vi "BRig_RT__Case_Exp__State_WrongOrTimeout_Pre__v11.vi"(0 "input_dataCurrent":u16[](array[numeric]), 5 "input_WorTO":bool, 6 "input_dataLC":u16[](array[numeric]), 7 "input_dataBlock":u16[][](array[numeric]), 9 "input_dataTrial":u16[][](array[numeric]), 11 "input_dataExp":u16[](array[numeric])) -> (1 "output_BTPR":bool, 2 "output_T2R":bool, 3 "output_T2R_or_BTPR":u16, 4 "output_dataCurrent":u16[](array[numeric]), 8 "output_dataBlock":u16[][](array[numeric]), 10 "output_dataTrial":u16[][](array[numeric]), 12 "output_BTPRavg":dbl, 13 "output_T2Ravg":dbl, 14 "output_R(F)_or_L(T)":bool, 15 "output_haveNewAvg":bool)   [LabVIEW 2014]
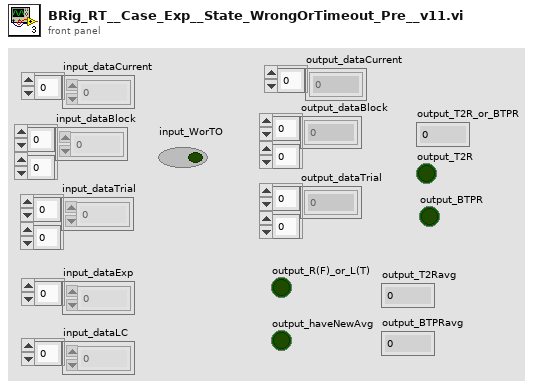
[diagram p1: front panel]
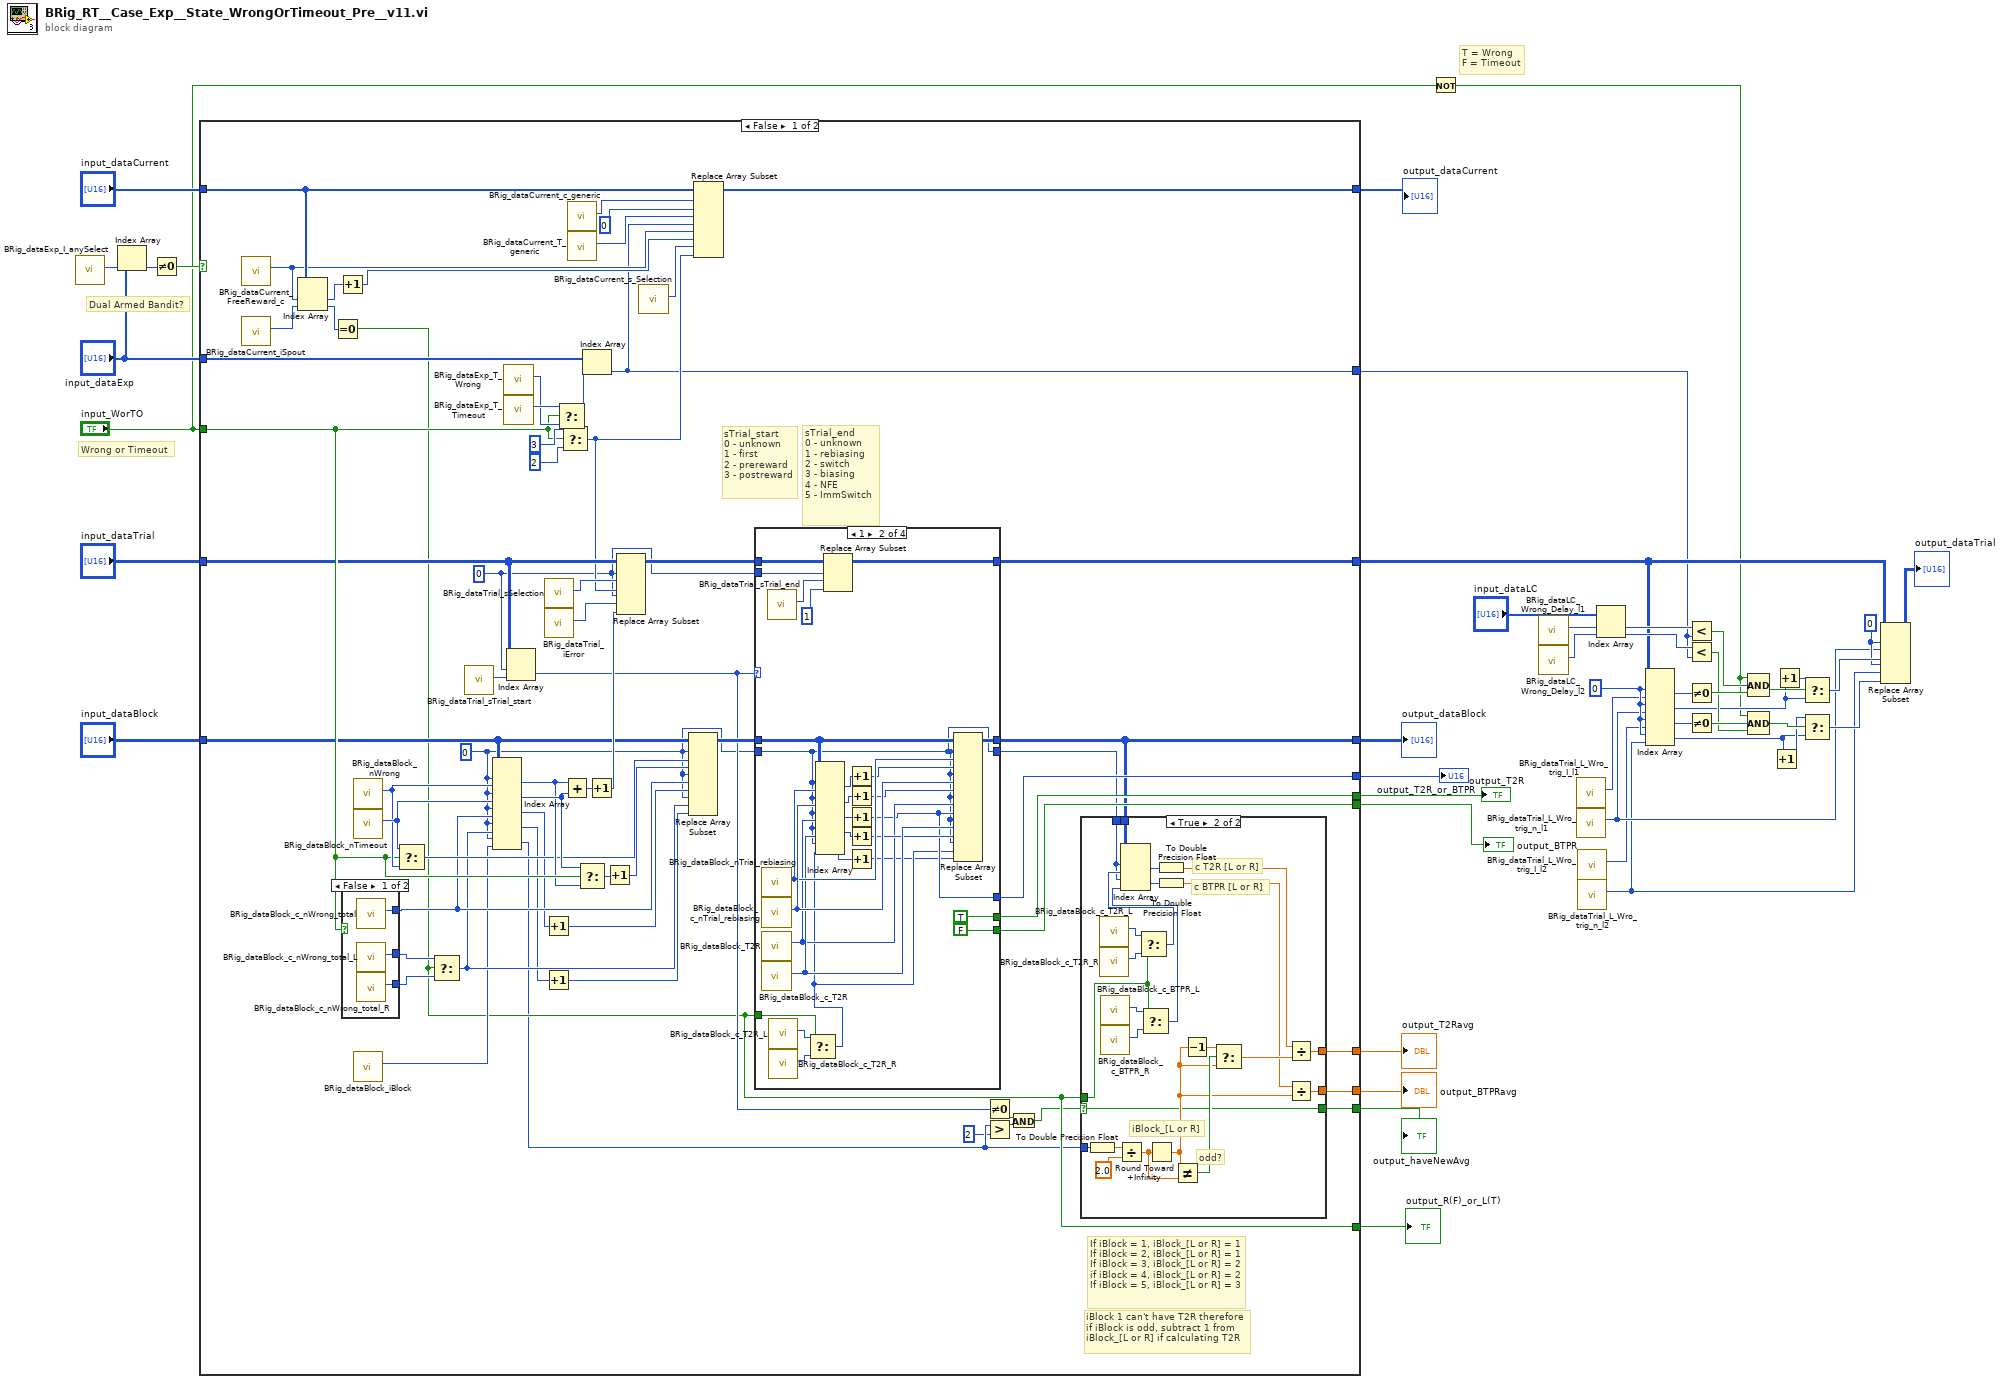
[diagram p0: block diagram]
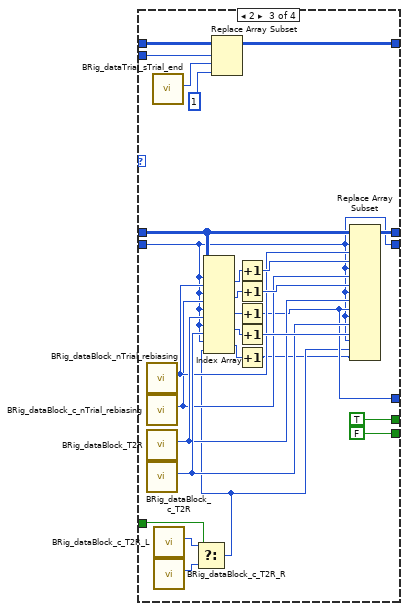
[diagram p4: hidden frame]
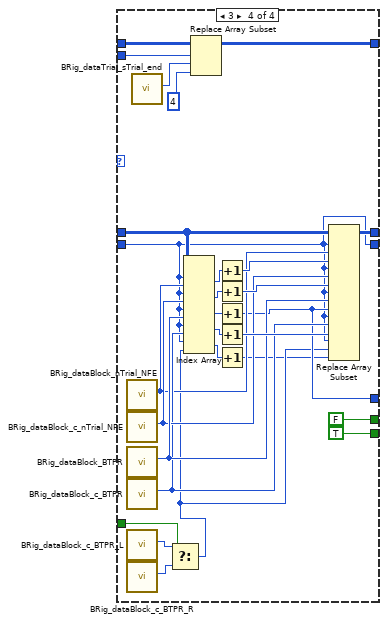
[diagram p5: hidden frame]
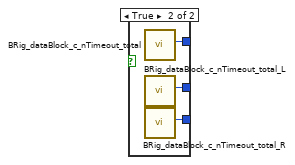
[diagram p6: hidden frame]
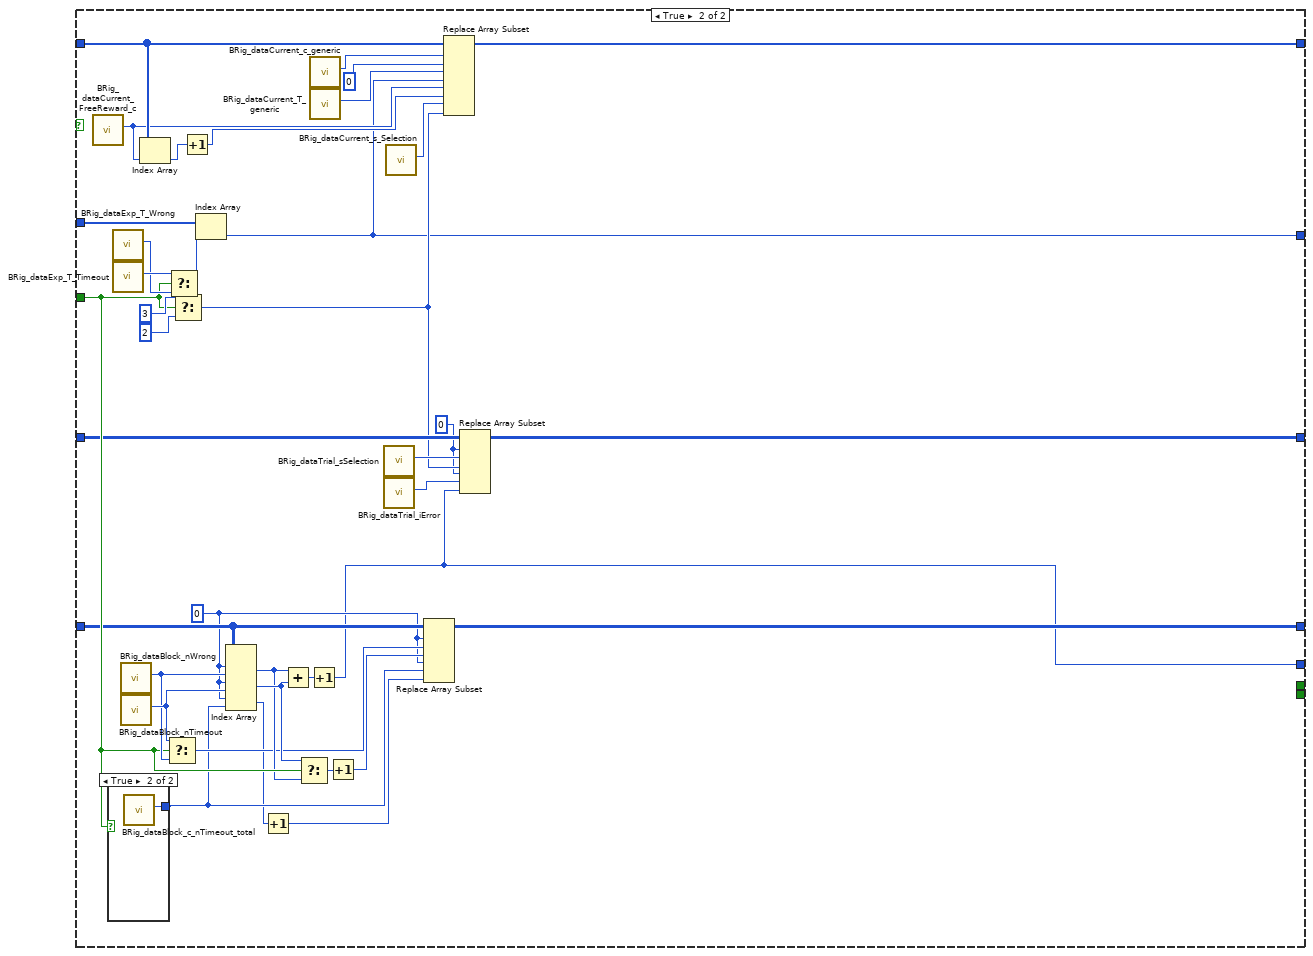
[diagram p7: hidden frame]
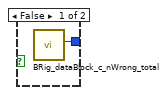
[diagram p8: hidden frame]
diagram:
  w17 = 0 ("index (row)")
  w27 = 0 ("disabled index (row)")
  # "T = Wrong\nF = Timeout"
  # "Wrong or Timeout"
  # "Dual Armed Bandit?"
  n1 = call "BRig_dataExp_I_anySelect.vi"() -> ("output_I_anySelect"=w34:i32)  [unwired: 11 in]
  n2 = Index Array(array="input_dataExp", index=w34) -> (element=w33:u16)
  n3 = Not Equal To 0?(x=w33) -> (x != 0?=w31:bool)
  n4 = case shown="False" w31 {
    tunnel: [w109 w264] -> w46
    tunnel: "input_dataCurrent" -> [w105 w260]
    tunnel: "input_dataExp" -> [w104 w259]
    tunnel: "input_WorTO" -> [w90 w248]
    tunnel: "input_dataBlock" -> [w86 w244]
    tunnel: "input_dataTrial" -> [w76 w238]
    tunnel: [w73 w231] -> w11
    tunnel: [w67 w228] -> w42
    tunnel: [w66 _] -> w41
    tunnel: [w65 _] -> w40
    tunnel: [w58 _] -> w39
    tunnel: [w57 w230] -> w38
    tunnel: [w55 _] -> w37
    tunnel: [w54 _] -> w36
    tunnel: [w53 _] -> w35
    tunnel: [w47 w227] -> w9
    frame False {
      w61 = 0
      w62 = 0
      # "iBlock 1 can't have T2R therefore\nif iBlock is odd, subtract 1 from\niBlock_[L or R] if calculating T2R"
      # "If iBlock = 1, iBlock_[L or R] = 1\nIf iBlock = 2, iBlock_[L or R] = 1\nIf iBlock = 3, iBlock_[L or R] = 2\nif iBlock = 4, iBlock_[L or R] = 2\nIf iBlock = 5, iBlock_[L or R] = 3"
      # "sTrial_end\n0 - unknown\n1 - rebiasing\n2 - switch\n3 - biasing\n4 - NFE\n5 - ImmSwitch"
      # "sTrial_start\n0 - unknown\n1 - first\n2 - prereward\n3 - postreward"
      n5 = call "BRig_dataCurrent_FreeReward_c.vi"() -> ("output_FreeReward_c"=w71:i32)  [unwired: 11 in]
      n6 = call "BRig_dataCurrent_iSpout.vi"() -> ("output_iSpout"=w60:i32)  [unwired: 11 in]
      n7 = Index Array(array=w105, index #1=w71, index #2=w60) -> (element #1=w72:u16, element #2=w59:u16)
      n8 = Equal To 0?(x=w59) -> (x = 0?=w58:bool)
      n9 = Increment(x=w72) -> (x+1=w70:u16)
      n10 = case shown="False" w90 {
        tunnel: [w223 w226] -> w83
        tunnel: [w222 w225] -> w96
        tunnel: [w221 w224] -> w95
        frame False {
          n11 = call "BRig_dataBlock_c_nWrong_total.vi"() -> ("output_c_nWrong_total"=w223:i32)  [unwired: 11 in]
          n12 = call "BRig_dataBlock_c_nWrong_total_L.vi"() -> ("output_c_nWrong_total_L"=w222:i32)  [unwired: 11 in]
          n13 = call "BRig_dataBlock_c_nWrong_total_R.vi"() -> ("output_c_nWrong_total_R"=w221:i32)  [unwired: 11 in]
        }
        frame True {
          n14 = call "BRig_dataBlock_c_nTimeout_total.vi"() -> ("output_c_nTimeout_total"=w226:i32)  [unwired: 11 in]
          n15 = call "BRig_dataBlock_c_nTimeout_total_L.vi"() -> ("output_c_nTimeout_total_L"=w225:i32)  [unwired: 11 in]
          n16 = call "BRig_dataBlock_c_nTimeout_total_R.vi"() -> ("output_c_nTimeout_total_R"=w224:i32)  [unwired: 11 in]
        }
      }
      n17 = call "BRig_dataBlock_nWrong.vi"() -> ("output_nWrong"=w91:i32)  [unwired: 11 in]
      n18 = call "BRig_dataBlock_nTimeout.vi"() -> ("output_nTimeout"=w92:i32)  [unwired: 11 in]
      n19 = call "BRig_dataBlock_iBlock.vi"() -> ("output_iBlock"=w64:i32)  [unwired: 11 in]
      n20 = Select(t=w92, s=w90, f=w91) -> (s? t:f=w85:i32)
      n21 = Select(t=w96, s=w58, f=w95) -> (s? t:f=w82:i32)
      n22 = call "BRig_dataTrial_sTrial_start.vi"() -> ("output_sTrial_start"=w77:i32)  [unwired: 11 in]
      n23 = Index Array(array=w86, index (row) #1=w61, index (col) #1=w91, index (row) #2=w61, index (col) #2=w92, index (row) #3=w61, index (col) #3=w83, index (row) #4=w61, index (col) #4=w82, index (row) #5=w61, index (col) #5=w64) -> (element #1=w88:u16, element #2=w89:u16, element #3=w81:u16, element #4=w80:u16, element #5=w52:u16)
      n24 = call "BRig_dataExp_T_Wrong.vi"() -> ("output_T_Wrong"=w101:i32)  [unwired: 11 in]
      n25 = call "BRig_dataExp_T_Timeout.vi"() -> ("output_T_Timeout"=w102:i32)  [unwired: 11 in]
      n26 = Index Array(array=w76, index (row)=w62, index (col)=w77) -> (element=w63:u16)
      n27 = Increment(x=w81) -> (x+1=w79:u16)
      n28 = Increment(x=w80) -> (x+1=w78:u16)
      n29 = call "BRig_dataTrial_sSelection.vi"() -> ("output_sSelection"=w98:i32)  [unwired: 11 in]
      n30 = call "BRig_dataTrial_iError.vi"() -> ("output_iError"=w97:i32)  [unwired: 11 in]
      n31 = Select(t=w102, s=w90, f=w101) -> (s? t:f=w103:i32)
      n32 = Select(t=u16 3 ("new element/subarray"), s=w90, f=u16 2 ("new element/subarray")) -> (s? t:f=w68:u16)
      n33 = Add(x=w88, y=w89) -> (x+y=w94:u16)
      n34 = call "BRig_dataCurrent_c_generic.vi"() -> ("output_count_generic"=w108:i32)  [unwired: 11 in]
      n35 = call "BRig_dataCurrent_T_generic.vi"() -> ("output_T_generic"=w107:i32)  [unwired: 11 in]
      n36 = Select(t=w89, s=w90, f=w88) -> (s? t:f=w87:u16)
      n37 = Index Array(array=w104, index=w103) -> (element=w47:u16)
      n38 = Increment(x=w94) -> (x+1=w93:u16)
      n39 = Increment(x=w87) -> (x+1=w84:u16)
      n40 = Replace Array Subset(array=w76, new element #1=w68, index (row) #1=w62, index (col) #1=w98, new element #2=w93, index (row) #2=w62, index (col) #2=w97) -> (w75:u16[][])
      n41 = call "BRig_dataCurrent_s_Selection.vi"() -> ("output_s_Selection"=w69:i32)  [unwired: 11 in]
      n42 = Replace Array Subset(array=w86, new element #1=w84, index (row) #1=w61, index (col) #1=w85, new element #2=w79, index (row) #2=w61, index (col) #2=w83, new element #3=w78, index (row) #3=w61, index (col) #3=w82) -> (w74:u16[][])
      n43 = Replace Array Subset(array=w105, new element #1=u16 0 ("new element/subarray"), index #1=w108, new element #2=w47, index #2=w107, new element #3=w70, index #3=w71, new element #4=w68, index #4=w69) -> (w109:u16[])
      n44 = case shown="1" w63 {
        tunnel: w75 -> [w136 w164 w192 w220]
        tunnel: w62 -> [_ w162 w190 w218]
        tunnel: [w136 w163 w191 w219] -> w73
        tunnel: w74 -> [w135 w153 w176 w208]
        tunnel: [w135 w152 w175 w207] -> w57
        tunnel: w61 -> [w134 w137 w165 w193]
        tunnel: [_ w144 w174 w200] -> w67
        tunnel: [_ TRUE TRUE FALSE] -> w66
        tunnel: [_ FALSE FALSE TRUE] -> w65
        tunnel: w58 -> [_ w143 w167 w199]
        tunnel: [w134 w137 w165 w193] -> w56
        frame 0, Default {
        }
        frame 1 {
          n45 = call "BRig_dataBlock_nTrial_rebiasing.vi"() -> ("output_nTrial_rebiasing"=w158:i32)  [unwired: 11 in]
          n46 = call "BRig_dataBlock_c_nTrial_rebiasing.vi"() -> ("output_c_nTrial_rebiasing"=w159:i32)  [unwired: 11 in]
          n47 = call "BRig_dataBlock_T2R.vi"() -> ("output_T2R"=w147:i32)  [unwired: 11 in]
          n48 = call "BRig_dataBlock_c_T2R.vi"() -> ("output_c_T2R"=w149:i32)  [unwired: 11 in]
          n49 = call "BRig_dataTrial_sTrial_end.vi"() -> ("output_sTrial_end"=w161:i32)  [unwired: 11 in]
          n50 = call "BRig_dataBlock_c_T2R_L.vi"() -> ("output_c_T2R_L"=w142:i32)  [unwired: 11 in]
          n51 = call "BRig_dataBlock_c_T2R_R.vi"() -> ("output_c_T2R_R"=w141:i32)  [unwired: 11 in]
          n52 = Select(t=w142, s=w143, f=w141) -> (s? t:f=w139:i32)
          n53 = Index Array(array=w153, index (row) #1=w137, index (col) #1=w158, index (row) #2=w137, index (col) #2=w159, index (row) #3=w137, index (col) #3=w147, index (row) #4=w137, index (col) #4=w149, index (row) #5=w137, index (col) #5=w139) -> (element #1=w157:u16, element #2=w155:u16, element #3=w151:u16, element #4=w150:u16, element #5=w140:u16)
          n54 = Replace Array Subset(array=w164, new element=u16 1 ("new element/subarray"), index (row)=w162, index (col)=w161) -> (w163:u16[][])
          n55 = Increment(x=w157) -> (x+1=w156:u16)
          n56 = Increment(x=w155) -> (x+1=w154:u16)
          n57 = Increment(x=w151) -> (x+1=w144:u16)
          n58 = Increment(x=w150) -> (x+1=w148:u16)
          n59 = Increment(x=w140) -> (x+1=w138:u16)
          n60 = Replace Array Subset(array=w153, new element #1=w156, index (row) #1=w137, index (col) #1=w158, new element #2=w154, index (row) #2=w137, index (col) #2=w159, new element #3=w144, index (row) #3=w137, index (col) #3=w147, new element #4=w148, index (row) #4=w137, index (col) #4=w149, new element #5=w138, index (row) #5=w137, index (col) #5=w139) -> (w152:u16[][])
        }
        frame 2 {
          n61 = call "BRig_dataBlock_nTrial_rebiasing.vi"() -> ("output_nTrial_rebiasing"=w178:i32)  [unwired: 11 in]
          n62 = call "BRig_dataBlock_c_nTrial_rebiasing.vi"() -> ("output_c_nTrial_rebiasing"=w177:i32)  [unwired: 11 in]
          n63 = call "BRig_dataBlock_T2R.vi"() -> ("output_T2R"=w185:i32)  [unwired: 11 in]
          n64 = call "BRig_dataBlock_c_T2R.vi"() -> ("output_c_T2R"=w186:i32)  [unwired: 11 in]
          n65 = call "BRig_dataTrial_sTrial_end.vi"() -> ("output_sTrial_end"=w189:i32)  [unwired: 11 in]
          n66 = call "BRig_dataBlock_c_T2R_L.vi"() -> ("output_c_T2R_L"=w171:i32)  [unwired: 11 in]
          n67 = call "BRig_dataBlock_c_T2R_R.vi"() -> ("output_c_T2R_R"=w170:i32)  [unwired: 11 in]
          n68 = Select(t=w171, s=w167, f=w170) -> (s? t:f=w168:i32)
          n69 = Index Array(array=w176, index (row) #1=w165, index (col) #1=w178, index (row) #2=w165, index (col) #2=w177, index (row) #3=w165, index (col) #3=w185, index (row) #4=w165, index (col) #4=w186, index (row) #5=w165, index (col) #5=w168) -> (element #1=w179:u16, element #2=w181:u16, element #3=w183:u16, element #4=w184:u16, element #5=w169:u16)
          n70 = Replace Array Subset(array=w192, new element=u16 1 ("new element/subarray"), index (row)=w190, index (col)=w189) -> (w191:u16[][])
          n71 = Increment(x=w179) -> (x+1=w180:u16)
          n72 = Increment(x=w181) -> (x+1=w182:u16)
          n73 = Increment(x=w183) -> (x+1=w174:u16)
          n74 = Increment(x=w184) -> (x+1=w187:u16)
          n75 = Increment(x=w169) -> (x+1=w166:u16)
          n76 = Replace Array Subset(array=w176, new element #1=w180, index (row) #1=w165, index (col) #1=w178, new element #2=w182, index (row) #2=w165, index (col) #2=w177, new element #3=w174, index (row) #3=w165, index (col) #3=w185, new element #4=w187, index (row) #4=w165, index (col) #4=w186, new element #5=w166, index (row) #5=w165, index (col) #5=w168) -> (w175:u16[][])
        }
        frame 3 {
          n77 = call "BRig_dataBlock_nTrial_NFE.vi"() -> ("output_nTrial_NFE"=w203:i32)  [unwired: 11 in]
          n78 = call "BRig_dataBlock_c_nTrial_NFE.vi"() -> ("output_c_nTrial_NFE"=w205:i32)  [unwired: 11 in]
          n79 = call "BRig_dataBlock_BTPR.vi"() -> ("output_BTPR"=w206:i32)  [unwired: 11 in]
          n80 = call "BRig_dataBlock_c_BTPR.vi"() -> ("output_c_BTPR"=w204:i32)  [unwired: 11 in]
          n81 = call "BRig_dataBlock_c_BTPR_L.vi"() -> ("output_c_BTPR_L"=w198:i32)  [unwired: 11 in]
          n82 = call "BRig_dataBlock_c_BTPR_R.vi"() -> ("output_c_BTPR_R"=w197:i32)  [unwired: 11 in]
          n83 = call "BRig_dataTrial_sTrial_end.vi"() -> ("output_sTrial_end"=w217:i32)  [unwired: 11 in]
          n84 = Select(t=w198, s=w199, f=w197) -> (s? t:f=w195:i32)
          n85 = Index Array(array=w208, index (row) #1=w193, index (col) #1=w203, index (row) #2=w193, index (col) #2=w205, index (row) #3=w193, index (col) #3=w206, index (row) #4=w193, index (col) #4=w204, index (row) #5=w193, index (col) #5=w195) -> (element #1=w209:u16, element #2=w211:u16, element #3=w213:u16, element #4=w214:u16, element #5=w196:u16)
          n86 = Replace Array Subset(array=w220, new element=u16 4 ("new element/subarray"), index (row)=w218, index (col)=w217) -> (w219:u16[][])
          n87 = Increment(x=w209) -> (x+1=w210:u16)
          n88 = Increment(x=w211) -> (x+1=w212:u16)
          n89 = Increment(x=w213) -> (x+1=w200:u16)
          n90 = Increment(x=w214) -> (x+1=w215:u16)
          n91 = Increment(x=w196) -> (x+1=w194:u16)
          n92 = Replace Array Subset(array=w208, new element #1=w210, index (row) #1=w193, index (col) #1=w203, new element #2=w212, index (row) #2=w193, index (col) #2=w205, new element #3=w200, index (row) #3=w193, index (col) #3=w206, new element #4=w215, index (row) #4=w193, index (col) #4=w204, new element #5=w194, index (row) #5=w193, index (col) #5=w195) -> (w207:u16[][])
        }
      }
      n93 = Not Equal To 0?(x=w63) -> (x != 0?=w49:bool)
      n94 = Greater?(x=w52, y=u16 2) -> (0:w50:bool)
      n95 = And(x=w49, y=w50) -> (x .and. y?=w48:bool)
      n96 = case shown="True" w48 {
        selector: w48 -> [_ w110]
        tunnel: w58 -> [_ w125]
        tunnel: w57 -> [_ w128]
        tunnel: w56 -> [_ w127]
        tunnel: w52 -> [_ w121]
        tunnel: [_ w112] -> w55
        tunnel: [_ w111] -> w54
        tunnel: [_ w110] -> w53
        frame False {
        }
        frame True {
          # "c BTPR [L or R]"
          # "c T2R [L or R]"
          # "odd?"
          # "iBlock_[L or R]"
          n97 = To Double Precision Float(number=w121) -> (double precision float=w124:dbl)
          n98 = call "BRig_dataBlock_c_T2R_L.vi"() -> ("output_c_T2R_L"=w132:i32)  [unwired: 11 in]
          n99 = call "BRig_dataBlock_c_T2R_R.vi"() -> ("output_c_T2R_R"=w133:i32)  [unwired: 11 in]
          n100 = call "BRig_dataBlock_c_BTPR_L.vi"() -> ("output_c_BTPR_L"=w130:i32)  [unwired: 11 in]
          n101 = call "BRig_dataBlock_c_BTPR_R.vi"() -> ("output_c_BTPR_R"=w131:i32)  [unwired: 11 in]
          n102 = Divide(x=w124, y=2.0) -> (x/y=w122:dbl)
          n103 = Select(t=w132, s=w125, f=w133) -> (s? t:f=w129:i32)
          n104 = Select(t=w130, s=w125, f=w131) -> (s? t:f=w126:i32)
          n105 = Index Array(array=w128, index (row) #1=w127, index (col) #1=w129, index (row) #2=w127, index (col) #2=w126) -> (element #1=w116:u16, element #2=w117:u16)
          n106 = Round Toward +Infinity(x=w122) -> (ceil(x): smallest int >= x=w115:dbl)
          n107 = To Double Precision Float(number=w116) -> (double precision float=w114:dbl)
          n108 = To Double Precision Float(number=w117) -> (double precision float=w113:dbl)
          n109 = Not Equal?(x=w115, y=w122) -> (x != y?=w119:bool)
          n110 = Decrement(x=w115) -> (x-1=w120:dbl)
          n111 = Select(t=w120, s=w119, f=w115) -> (s? t:f=w118:dbl)
          n112 = Divide(x=w114, y=w118) -> (x/y=w112:dbl)
          n113 = Divide(x=w113, y=w115) -> (x/y=w111:dbl)
        }
      }
    }
    frame True {
      w229 = 0
      w232 = 0
      n114 = call "BRig_dataCurrent_FreeReward_c.vi"() -> ("output_FreeReward_c"=w236:i32)  [unwired: 11 in]
      n115 = case shown="True" w248 {
        tunnel: [w265 w266] -> w241
        frame False {
          n116 = call "BRig_dataBlock_c_nWrong_total.vi"() -> ("output_c_nWrong_total"=w265:i32)  [unwired: 11 in]
        }
        frame True {
          n117 = call "BRig_dataBlock_c_nTimeout_total.vi"() -> ("output_c_nTimeout_total"=w266:i32)  [unwired: 11 in]
        }
      }
      n118 = call "BRig_dataExp_T_Wrong.vi"() -> ("output_T_Wrong"=w256:i32)  [unwired: 11 in]
      n119 = call "BRig_dataExp_T_Timeout.vi"() -> ("output_T_Timeout"=w257:i32)  [unwired: 11 in]
      n120 = call "BRig_dataBlock_nWrong.vi"() -> ("output_nWrong"=w249:i32)  [unwired: 11 in]
      n121 = call "BRig_dataBlock_nTimeout.vi"() -> ("output_nTimeout"=w250:i32)  [unwired: 11 in]
      n122 = Index Array(array=w260, index=w236) -> (element=w237:u16)
      n123 = Select(t=w250, s=w248, f=w249) -> (s? t:f=w243:i32)
      n124 = Select(t=w257, s=w248, f=w256) -> (s? t:f=w258:i32)
      n125 = Select(t=u16 3 ("new element/subarray"), s=w248, f=u16 2 ("new element/subarray")) -> (s? t:f=w233:u16)
      n126 = Increment(x=w237) -> (x+1=w235:u16)
      n127 = Index Array(array=w259, index=w258) -> (element=w227:u16)
      n128 = Index Array(array=w244, index (row) #1=w229, index (col) #1=w249, index (row) #2=w229, index (col) #2=w250, index (row) #3=w229, index (col) #3=w241) -> (element #1=w246:u16, element #2=w247:u16, element #3=w240:u16)
      n129 = Increment(x=w240) -> (x+1=w239:u16)
      n130 = Add(x=w246, y=w247) -> (x+y=w251:u16)
      n131 = Select(t=w247, s=w248, f=w246) -> (s? t:f=w245:u16)
      n132 = Increment(x=w251) -> (x+1=w228:u16)
      n133 = call "BRig_dataCurrent_c_generic.vi"() -> ("output_count_generic"=w263:i32)  [unwired: 11 in]
      n134 = call "BRig_dataCurrent_T_generic.vi"() -> ("output_T_generic"=w262:i32)  [unwired: 11 in]
      n135 = Increment(x=w245) -> (x+1=w242:u16)
      n136 = call "BRig_dataTrial_sSelection.vi"() -> ("output_sSelection"=w253:i32)  [unwired: 11 in]
      n137 = call "BRig_dataTrial_iError.vi"() -> ("output_iError"=w252:i32)  [unwired: 11 in]
      n138 = call "BRig_dataCurrent_s_Selection.vi"() -> ("output_s_Selection"=w234:i32)  [unwired: 11 in]
      n139 = Replace Array Subset(array=w244, new element #1=w242, index (row) #1=w229, index (col) #1=w243, new element #2=w239, index (row) #2=w229, index (col) #2=w241) -> (w230:u16[][])
      n140 = Replace Array Subset(array=w260, new element #1=u16 0 ("new element/subarray"), index #1=w263, new element #2=w227, index #2=w262, new element #3=w235, index #3=w236, new element #4=w233, index #4=w234) -> (w264:u16[])
      n141 = Replace Array Subset(array=w238, new element #1=w233, index (row) #1=w232, index (col) #1=w253, new element #2=w228, index (row) #2=w232, index (col) #2=w252) -> (w231:u16[][])
    }
  }
  "output_dataCurrent" <- w46
  "output_dataBlock" <- w38
  "output_T2R_or_BTPR" <- w42
  "output_T2R" <- w41
  "output_BTPR" <- w40
  "output_R(F)_or_L(T)" <- w39
  "output_T2Ravg" <- w37
  "output_BTPRavg" <- w36
  "output_haveNewAvg" <- w35
  n142 = Not(x="input_WorTO") -> (.not. x?=w7:bool)
  n143 = call "BRig_dataLC_Wrong_Delay_l1.vi"() -> ("output_Wrong_Delay"=w5:i32)  [unwired: 11 in]
  n144 = call "BRig_dataLC_Wrong_Delay_l2.vi"() -> ("output_Wrong_Delay_l2"=w6:i32)  [unwired: 11 in]
  n145 = call "BRig_dataTrial_L_Wro_trig_I_l1.vi"() -> ("output_L_Wro_trig_I_l1"=w4:i32)  [unwired: 11 in]
  n146 = call "BRig_dataTrial_L_Wro_trig_n_l1.vi"() -> ("output_L_Wrong_trig_n_l1"=w3:i32)  [unwired: 11 in]
  n147 = call "BRig_dataTrial_L_Wro_trig_I_l2.vi"() -> ("output_L_Wro_trig_I_l2"=w2:i32)  [unwired: 11 in]
  n148 = call "BRig_dataTrial_L_Wro_trig_n_l2.vi"() -> ("output_L_Wrong_trig_n_l2"=w1:i32)  [unwired: 11 in]
  n149 = Index Array(array="input_dataLC", index #1=w5, index #2=w6) -> (element #1=w30:u16, element #2=w29:u16)
  n150 = Index Array(array=w11, index (row) #1=w27, index (col) #1=w4, index (row) #2=w27, index (col) #2=w3, index (row) #3=w27, index (col) #3=w2, index (row) #4=w27, index (col) #4=w1) -> (element #1=w28:u16, element #2=w19:u16, element #3=w26:u16, element #4=w14:u16)
  n151 = Less?(x=w30, y=w9) -> (x < y?=w24:bool)
  n152 = Less?(x=w29, y=w9) -> (x < y?=w22:bool)
  n153 = Not Equal To 0?(x=w28) -> (x != 0?=w25:bool)
  n154 = Not Equal To 0?(x=w26) -> (x != 0?=w23:bool)
  n155 = Compound Arithmetic op=AND(w7, w24, w25) -> (w21:bool)
  n156 = Compound Arithmetic op=AND(w7, w23, w22) -> (w16:bool)
  n157 = Increment(x=w14) -> (x+1=w15:u16)
  n158 = Increment(x=w19) -> (x+1=w20:u16)
  n159 = Select(t=w20, s=w21, f=w19) -> (s? t:f=w18:u16)
  n160 = Select(t=w15, s=w16, f=w14) -> (s? t:f=w13:u16)
  n161 = Replace Array Subset(array=w11, new element #1=w18, index (row) #1=w17, index (col) #1=w3, new element #2=w13, index (row) #2=w17, index (col) #2=w1) -> (→"output_dataTrial":u16[][])
